vi "DMM_Resistance Meas Configure and Measure.vi"(0 "DMM Handle In":refnum<k15>, 2 "Execution Option":T8, 5 "Function Settings":T6={"Range and Function"=enum."2w-Resistance Auto Range", "Resolution in Digits"=5.5} {"Resolution in Digits" items=["3 1/2"=3.5, "4 1/2"=4.5, "5 1/2"=5.5, "6 1/2"=6.5, "7 1/2"=7.5]}, 7 "Timing and Trigger Settings":T3={"Aperture Time (s)"=-1.0, "Settle Time (s)"=-1.0, "Trigger Settings"={"Trigger Delay (sec)"=-1.0, "Enable Trigger?"=FALSE, "Trigger Source"=enum."Immediate", "Slope"=enum."Rising Edge"}} {"Trigger Settings"."Trigger Delay (sec)" format="%.4f"; "Aperture Time (s)" format="%#.6g"}, 11 "error in":errorcluster) -> (4 "DMM Handle Out":refnum<k15>, 6 "Measurement":T1={"Measured Value"=0.0, "Out of Range"=FALSE, "Unit"="Ohm", "Measurement"="0.0000Ohm"} {"Measured Value" format="%^#_9e"}, 8 "DMM Execution Settings":T2={"Absolute\nResolution"=0.0, "Input Resistance\n(Ohm)"=0.0, "Digits\nResolution"=0.0, "Range"=0.0, "Minimum\nFrequency (Hz)"=0.0, "Aperture\nTime (s)"=0.0, "Auto Range\nValue"=0.0, "Settle\nTime (s)"=0.0, "Function"=5} {"Function" items=["DC Volts"=1, "AC Volts"=2, "DC Current"=3, "AC Current"=4, "2-Wire Resistance"=5, "4-Wire Resistance"=101, "Frequency"=104, "Period"=105, "AC Volts DC Coupled"=1001, "Diode"=1002, "Waveform Voltage"=1003, "Waveform Current"=1004, "Capacitance"=1005, "Inductance"=1006, "Temperature"=108]; "Absolute\nResolution" format="%#_6p"; "Input Resistance\n(Ohm)" format="%#_6p"; "Range" format="%#_6p"; "Minimum\nFrequency (Hz)" format="%#_6p"; "Aperture\nTime (s)" format="%#_6p"; "Auto Range\nValue" format="%#_6p"; "Settle\nTime (s)" format="%#_6p"}, 15 "error out":errorcluster)   [LabVIEW 2021, in "DMM_Resistance Measurement.lvlib"]
doc: "Configures an NI-DMM 2-wire or 4-wire resistance measurement on the resource provided by the DMM Handle In control according to the given Function, Execution, and Timing & Trigger settings, and then executes the measurement (by default).\n\nAdditionally users can choose to Configure Only without executing the measurement or Measure Only using the existing configuration."
uses:
  DMM_Resistance Measurement.lvlib
  Common/Typedefs/Execution Options - Measure.ctl
  DMM Resistance Typedefs/Function Settings.ctl
  <instrlib>/niDMM/nidmm.llb/niDMM Resolution in Digits.ctl
  DMM Resistance Typedefs/Timing & Trigger Settings.ctl
  <instrlib>/niDMM/nidmm.llb/niDMM Trigger.ctl
  <instrlib>/niDMM/nidmm.llb/niDMM Slope.ctl
  DMM Resistance Typedefs/DMM Execution Settings.ctl
  DMM Resistance Typedefs/Measurement.ctl
  <instrlib>/niDMM/nidmm.llb/niDMM Configure Measurement Digits.vi
panel:
  # "Inputs"
  # "Outputs"
  # "Execution Settings"
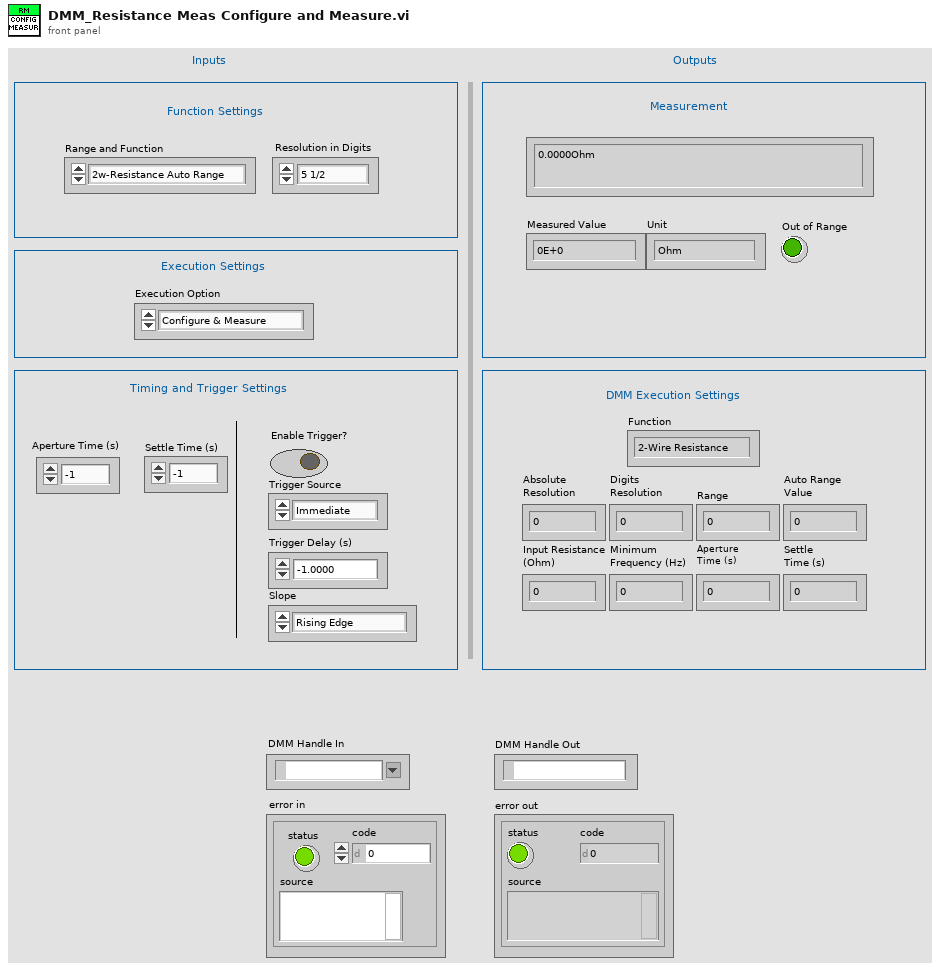
[diagram p1: front panel]
types:
  T1 = typedef "DMM_Resistance Measurement.lvlib/Measurement.ctl" = cluster{"Measured Value":dbl, "Out of Range":bool, "Unit":string, "Measurement":string}
  T2 = typedef "DMM_Resistance Measurement.lvlib/DMM Execution Settings.ctl" = cluster{"Absolute\nResolution":dbl, "Input Resistance\n(Ohm)":dbl, "Digits\nResolution":dbl, "Range":dbl, "Minimum\nFrequency (Hz)":dbl, "Aperture\nTime (s)":dbl, "Auto Range\nValue":dbl, "Settle\nTime (s)":dbl, "Function":i32}
  T3 = typedef "DMM_Resistance Measurement.lvlib/Timing & Trigger Settings.ctl" = cluster{"Aperture Time (s)":dbl, "Settle Time (s)":dbl, "Trigger Settings":cluster{"Trigger Delay (sec)":dbl, "Enable Trigger?":bool, "Trigger Source":T4, "Slope":T5}}
  T4 = typedef "niDMM Trigger.ctl" = enum16{"Immediate", "External", "TTL 0", "TTL 1", "TTL 2", "TTL 3", "TTL 4", "TTL 5", "TTL 6", "Software", "TTL 7", "PXI Star", "LBR Trig 1", "Aux Trig 1"}
  T5 = typedef "niDMM Slope.ctl" = enum16{"Rising Edge", "Falling Edge"}
  T6 = typedef "DMM_Resistance Measurement.lvlib/Function Settings.ctl" = cluster{"Range and Function":enum16{"2w-Resistance Auto Range", "2w-Res 100 Ohm", "2w-Res 1 kOhm", "2w-Res 10 kOhm", "2w-Res 100 kOhm", "2w-Res 1 MOhm", "2w-Res 10 MOhm", "2w-Res 100 MOhm", "2w-Res 5 GOhm", "     ", "4w-Resistance Auto Range", "4w-Res 100 Ohm", "4w-Res 1 kOhm", "4w-Res 10 kOhm", "4w-Res 100 kOhm", "4w-Res 1 MOhm", "4w-Res 10 MOhm"}, "Resolution in Digits":T7}
  T7 = typedef "niDMM Resolution in Digits.ctl" = dbl
  T8 = typedef "Execution Options - Measure.ctl" = enum16{"Configure & Measure", "Configure only", "Measure only"}
  T9 = typedef "niDMM Function.ctl" = enum16{"DC Volts", "AC Volts", "DC Current", "AC Current", "2-wire Resistance", "4-wire Resistance", "Diode", "Frequency", "Period", "AC Volts DC Coupled", "Capacitance", "Inductance", "Temperature"}
  T10 = cluster{"Range":dbl, "Function":T9, "AC Range":dbl, "Resolution in Digits":T7}
  T11 = cluster{"Trigger Delay (sec)":dbl, "Enable Trigger?":bool, "Trigger Source":T4, "Slope":T5}
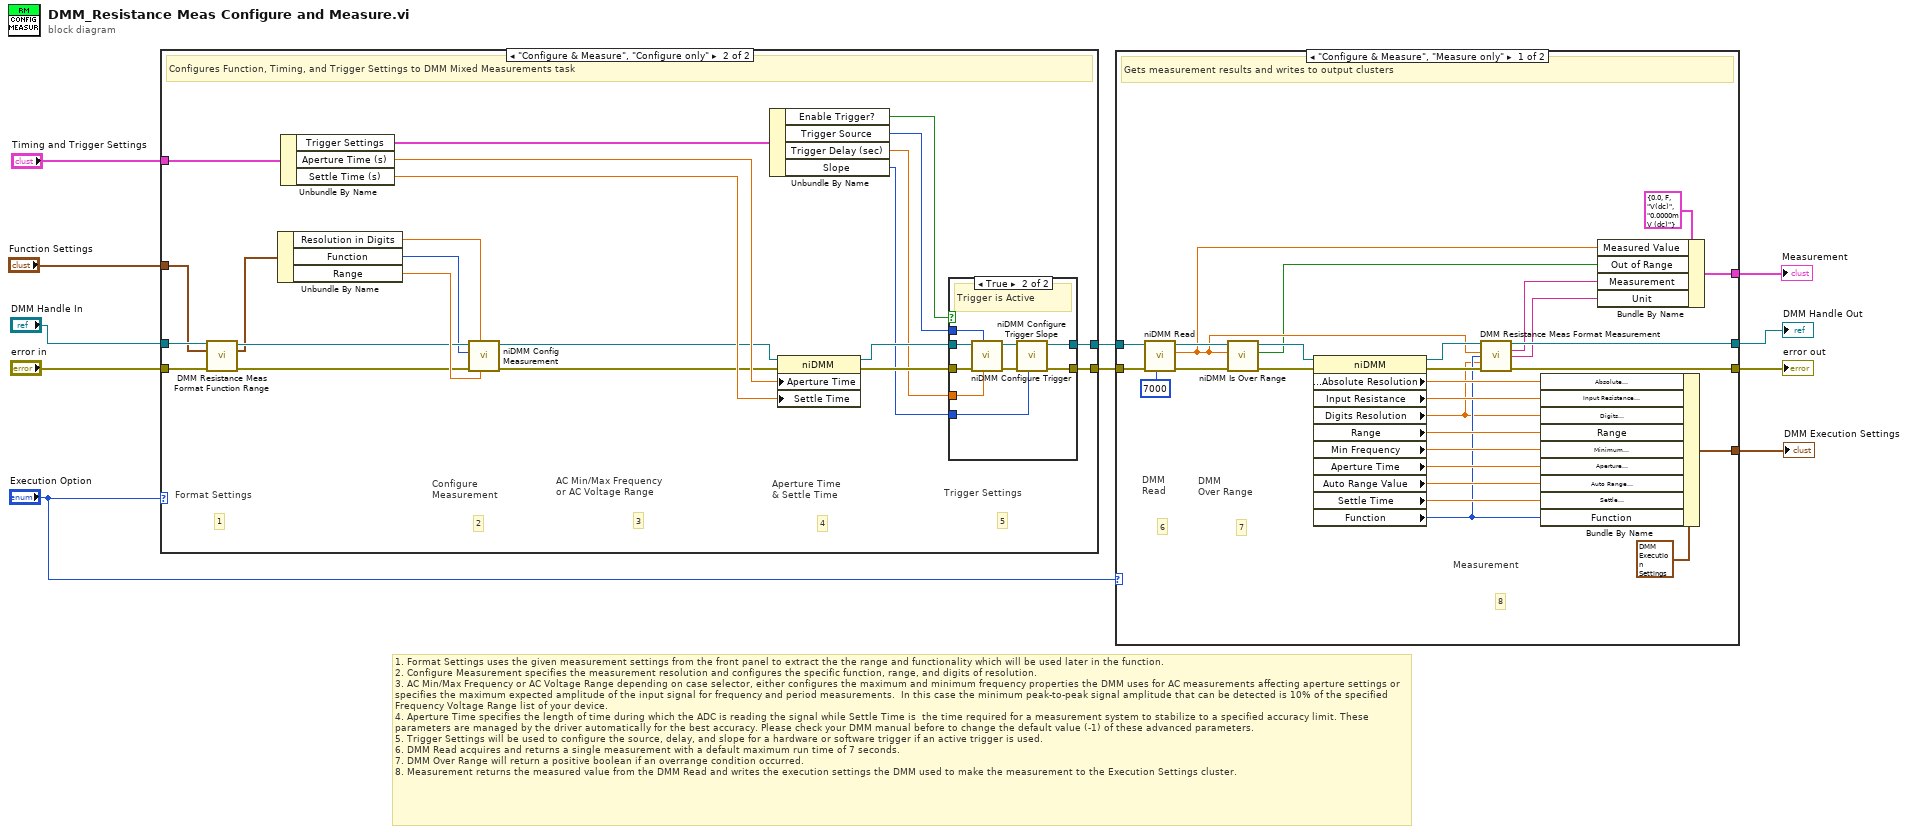
[diagram p0: block diagram]
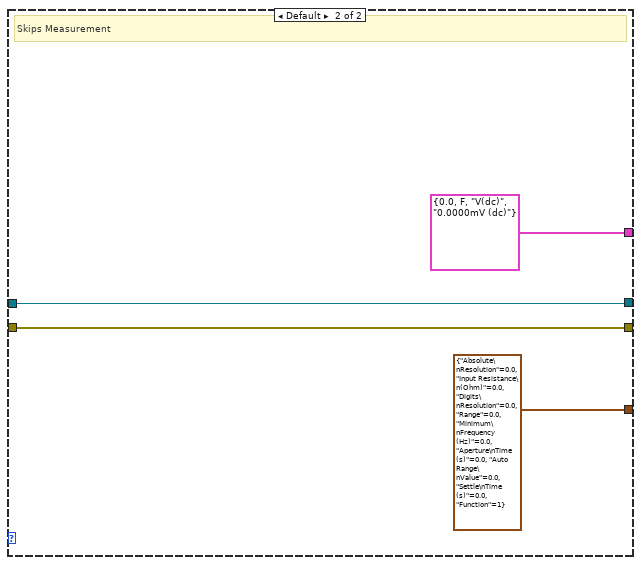
[diagram p2: hidden frame]
diagram:
  # "1. Format Settings uses the given measurement settings from the front panel to extract the the range and functionality which will be used later in the function.\n2. Configure Measurement specifies the measurement resolution and configures the specific function, range, and digits of resolution.\n3. AC Min/Max Frequency or AC Voltage Range depending on case selector, either configures the maximum and minimum frequency properties the DMM uses for AC measurements affecting aperture settings or specifies the maximum expected amplitude of the input signal for frequency and period measurements.  In this case the minimum peak-to-peak signal amplitude that can be detected is 10% of the specified Frequency Voltage Range list of your device.\n4. Aperture Time specifies the length of time during which the ADC is reading the signal while Settle Time is  the time required for a measurement system to stabilize to a specified accuracy limit. These parameters are managed by the driver automatically for the best accuracy. Please check your DMM manual before to change the default value (-1) of these advanced parameters.\n5. Trigger Settings will be used to configure the source, delay, and slope for a hardware or software trigger if an active trigger is used.\n6. DMM Read acquires and returns a single measurement with a default maximum run time of 7 seconds.\n7. DMM Over Range will return a positive boolean if an overrange condition occurred.\n8. Measurement returns the measured value from the DMM Read and writes the execution settings the DMM used to make the measurement to the Execution Settings cluster."
  n1 = case shown="\"Configure & Measure\", \"Configure only\"" "Execution Option" {
    tunnel: [w13 w34] -> w11
    tunnel: [w12 w33] -> w10
    tunnel: "Timing and Trigger Settings" -> [_ w32]
    tunnel: "DMM Handle In" -> [w13 w22]
    tunnel: "Function Settings" -> [_ w16]
    tunnel: "error in" -> [w12 w20]
    frame "Measure only" {
      # "Skips Configurations (Function, Timing and Trigger Settings)"
    }
    frame "Configure & Measure", "Configure only" {
      # "4"
      # "Aperture Time \n& Settle Time"
      # "1"
      # "Format Settings"
      # "5"
      # "3"
      # "2"
      # "Configure\nMeasurement"
      # "Trigger Settings"
      # "AC Min/Max Frequency\nor AC Voltage Range"
      # "Configures Function, Timing, and Trigger Settings to DMM Mixed Measurements task"
      n2 = call "DMM Resistance Meas Format Function Range.vi"("DMM Handle In"=w22, "Function Settings In"=w16, "error in"=w20) -> ("DMM Handle Out"=w21:refnum<k15>, "Function Settings Out"=w18:T10, "error out"=w23:errorcluster)  [unwired: 10 in]
      n3 = Unbundle By Name(w18) -> ("Resolution in Digits"=w19:T7, "Function"=w17:T9, "Range"=w28:dbl)
      n4 = Unbundle By Name(w32) -> ("Trigger Settings"=w27:T11, "Aperture Time (s)"=w25:dbl, "Settle Time (s)"=w24:dbl)
      n5 = call-poly <instrlib>:"niDMM Config Measurement.vi"("Range"=w28, "Resolution in Digits"=w19, "error in (no error)"=w23, "Function"=w17, "instrument handle"=w21) -> ("error out"=w14:errorcluster, "instrument handle out"=w15:refnum<k15>)  [unwired: 5 in]
      n6 = Unbundle By Name(w27) -> ("Enable Trigger?"=w31:bool, "Trigger Source"=w30:T4, "Trigger Delay (sec)"=w29:dbl, "Slope"=w26:T5)
      n7 = property class="niDMM"(reference=w15, error in=w14, "Aperture Time"=w25, "Settle Time"=w24) -> (reference out=w35:refnum<k15>, error out=w36:errorcluster)
      n8 = case shown="True" w31 {
        tunnel: w36 -> [w37 w46]
        tunnel: w35 -> [w38 w47]
        tunnel: [w38 w41] -> w34
        tunnel: [w37 w40] -> w33
        tunnel: w30 -> [_ w44]
        tunnel: w29 -> [_ w45]
        tunnel: w26 -> [_ w39]
        frame False {
          # "No Trigger"
        }
        frame True {
          # "Trigger is Active"
          n9 = call <instrlib>:"niDMM Configure Trigger.vi"("Trigger Delay (sec)"=w45, "Trigger Source"=w44, "error in (no error)"=w46, "instrument handle"=w47) -> ("error out"=w43:errorcluster, "instrument handle out"=w42:refnum<k15>)  [unwired: 6 in]
          n10 = call <instrlib>:"niDMM Configure Trigger Slope.vi"("Slope"=w39, "error in (no error)"=w43, "instrument handle"=w42) -> ("error out"=w40:errorcluster, "instrument handle out"=w41:refnum<k15>)  [unwired: 7 in]
        }
      }
    }
  }
  n11 = case shown="\"Configure & Measure\", \"Measure only\"" "Execution Option" {
    tunnel: w11 -> [w75 w78]
    tunnel: w10 -> [w74 w79]
    tunnel: [w58 w78] -> w6
    tunnel: [w57 w79] -> w9
    tunnel: [w49 T2 {"Absolute\nResolution"=0.0, "Input Resistance\n(Ohm)"=0.0, "Digits\nResolution"=0.0, "Range"=0.0, "Minimum\nFrequency (Hz)"=0.0, "Aperture\nTime (s)"=0.0, "Auto Range\nValue"=0.0, "Settle\nTime (s)"=0.0, "Function"=1} ("Execution Settings 2")] -> w2
    tunnel: [w63 T1 {"Measured Value"=0.0, "Out of Range"=FALSE, "Unit"="V(dc)", "Measurement"="0.0000mV (dc)"}] -> w1
    frame "Configure & Measure", "Measure only" {
      # "7"
      # "DMM \nOver Range"
      # "6"
      # "DMM \nRead"
      # "8"
      # "Measurement"
      # "Gets measurement results and writes to output clusters"
      n12 = call <instrlib>:"niDMM Read.vi"("Maximum Time (msec)"=7000, "error in (no error)"=w74, "instrument handle"=w75) -> ("error out"=w72:errorcluster, "Measurement"=w52:dbl, "instrument handle out"=w73:refnum<k15>)  [unwired: 6 in]
      n13 = call <instrlib>:"niDMM Is Over Range.vi"("error in (no error)"=w72, "Measurement"=w52, "instrument handle"=w73) -> ("error out"=w70:errorcluster, "Over Range?"=w51:bool, "instrument handle out"=w71:refnum<k15>)  [unwired: 6 in]
      n14 = property class="niDMM"(reference=w71, error in=w70) -> (reference out=w60:refnum<k15>, error out=w59:errorcluster, "Configuration:Absolute Resolution"=w62:dbl, "Input Resistance"=w69:dbl, "Digits Resolution"=w53:dbl, "Range"=w68:dbl, "Min Frequency"=w67:dbl, "Aperture Time"=w66:dbl, "Auto Range Value"=w65:dbl, "Settle Time"=w64:dbl, "Function"=w54:i32)
      n15 = call "DMM Resistance Meas Format Measurement.vi"("DMM Handle In"=w60, "Measured Value"=w52, "Function"=w54, "Digits Resolution"=w53, "error in"=w59) -> ("DMM Handle Out"=w58:refnum<k15>, "Measurement"=w56:string, "Unit"=w55:string, "error out"=w57:errorcluster)  [unwired: 7 in]
      n16 = Bundle By Name(cluster=T2 {"Absolute\nResolution"=0.0, "Input Resistance\n(Ohm)"=0.0, "Digits\nResolution"=0.0, "Range"=0.0, "Minimum\nFrequency (Hz)"=0.0, "Aperture\nTime (s)"=0.0, "Auto Range\nValue"=0.0, "Settle\nTime (s)"=0.0, "Function"=1} ("Execution Settings"), "Absolute\nResolution"=w62, "Input Resistance\n(Ohm)"=w69, "Digits\nResolution"=w53, "Range"=w68, "Minimum\nFrequency (Hz)"=w67, "Aperture\nTime (s)"=w66, "Auto Range\nValue"=w65, "Settle\nTime (s)"=w64, "Function"=w54) -> (w49:T2)
      n17 = Bundle By Name(cluster=T1 {"Measured Value"=0.0, "Out of Range"=FALSE, "Unit"="V(dc)", "Measurement"="0.0000mV (dc)"}, "Measured Value"=w52, "Out of Range"=w51, "Measurement"=w56, "Unit"=w55) -> (w63:T1)
    }
    frame Default {
      # "Skips Measurement"
    }
  }
  "error out" <- w9
  "DMM Handle Out" <- w6
  "DMM Execution Settings" <- w2
  "Measurement" <- w1
